vi "GetType.vi"(8 "error in (no error)":errorcluster, 11 "Configure Thermocouple [TC] Msg":refnum<class "Configure Thermocouple [TC] Msg.lvclass">) -> (0 "error out":errorcluster, 2 "Data Sample":variant, 3 "Configure Thermocouple [TC] Msg":refnum<class "Configure Thermocouple [TC] Msg.lvclass">)   [LabVIEW 2016, in "CS++DMM.lvlib" / "Configure Thermocouple [TC] Msg.lvclass"]
uses:
  Configure Thermocouple [TC] Msg.lvclass
  Configure Thermocouple [TC] Msg.lvclass/Configure Thermocouple [TC] Msg.ctl
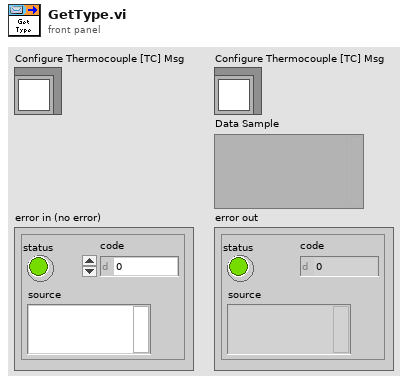
[diagram p1: front panel]
types:
  T1 = cluster{"thermocouple type (B)":i32, "ref junc type (Internal)":i32}
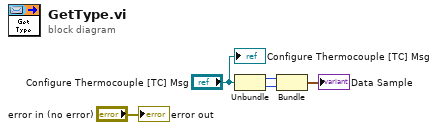
[diagram p0: block diagram]
diagram:
  n1 = Unbundle("Configure Thermocouple [TC] Msg") -> (w2:i32, w1:i32)
  n2 = Bundle("thermocouple type (B)"=w2, "ref junc type (Internal)"=w1) -> (→"Data Sample":T1)  [unwired: 1 in]
  "error out" <- "error in (no error)"
  "Configure Thermocouple [TC] Msg" <- "Configure Thermocouple [TC] Msg"
